vi "Variant to Class.vi"(8 "error in (no error)":errorcluster, 10 "Data in":variant, 11 "Run VI Node in":refnum<class "Run VI Node.lvclass">) -> (0 "error out":errorcluster, 2 "Data Out":variant, 3 "Run VI Node out":refnum<class "Run VI Node.lvclass">)   [LabVIEW 2014, in "Run VI Node.lvclass"]
uses:
  Run VI Node.lvclass
  Shared/Controls/Run VI - STYP.ctl
  Run VI Node.lvclass/Run VI Node.ctl
  Classes/Build Job/Build Job.lvclass
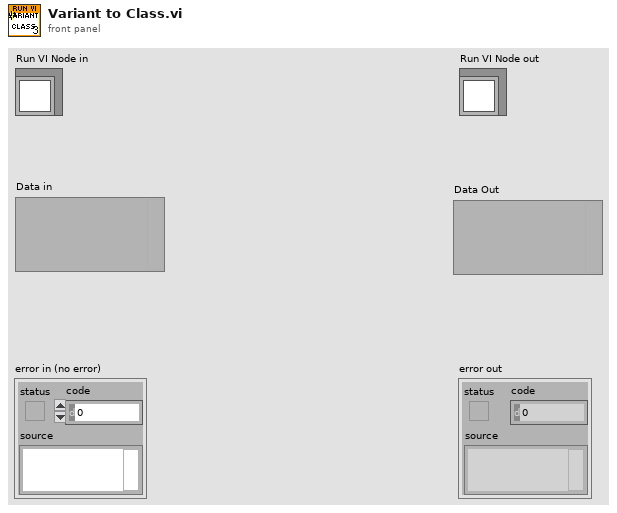
[diagram p1: front panel]
types:
  T1 = typedef "Run VI - STYP.ctl" = cluster{"Executor_Number":string, "VI_Path":string, "Wait_Until_Done":bool}
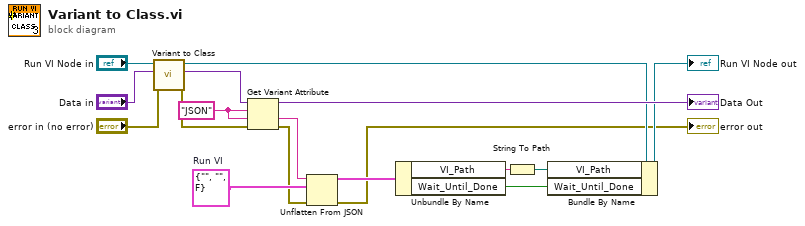
[diagram p0: block diagram]
diagram:
  w5 = T1 {"Executor_Number"="", "VI_Path"="", "Wait_Until_Done"=FALSE}  # Run VI
  w14 = "JSON" ("name")
  n1 = call-parent "Variant to Class.vi"("error in (no error)"="error in (no error)", "Data in"="Data in", "Build Job in"="Run VI Node in") -> ("error out"=w6:errorcluster, "Data Out"=w1:variant, "Build Job out"=w8:refnum<class "Run VI Node.lvclass">)  [unwired: 6 in]
  n2 = Get Variant Attribute(Variant=w1, name=w14, default value (empty Variant)=w14, error in=w6) -> (duplicate Variant=→"Data Out":variant, value=w13:string, error out=w3:errorcluster)  [unwired: 1 out]
  n3 = Unflatten From JSON(JSON string=w13, type and defaults=w5, error in (no error)=w3) -> (value=w12:T1, error out=→"error out":errorcluster)  [unwired: 4 in]
  n4 = Unbundle By Name(w12) -> ("VI_Path"=w11:string, "Wait_Until_Done"=w10:bool)
  n5 = String To Path(string=w11) -> (path=w4:path)
  n6 = Bundle By Name(cluster=w8, "VI_Path"=w4, "Wait_Until_Done"=w10) -> (→"Run VI Node out":refnum<class "Run VI Node.lvclass">)
